vi "4Bar Arm Control.vi"(8 "Enable Setup":bool, 9 "4Bar Button":bool, 10 "Disable Sensor":bool, 11 "Joystick Input":dbl) -> ()   [LabVIEW 2014]
panel:
  out "Pot Error Out":errorcluster
  out "In Range?":bool
  out "PID Output":dbl format="%.2f"
  out "Output to Motor":dbl
  in  "Height Above Ground":dbl(slide)=0.40816326530612246 scale=0.2..0.8
  in  "PID gains":T1={"proportional gain (Kc)"=25.0, "integral time (Ti, min)"=0.015, "derivative time (Td, min)"=0.0}
  out "4Bar Pot Value":dbl
  out "Motor Output 4Bar":dbl(slide) scale=-1.0..1.0
  out "Motor Error Out":errorcluster
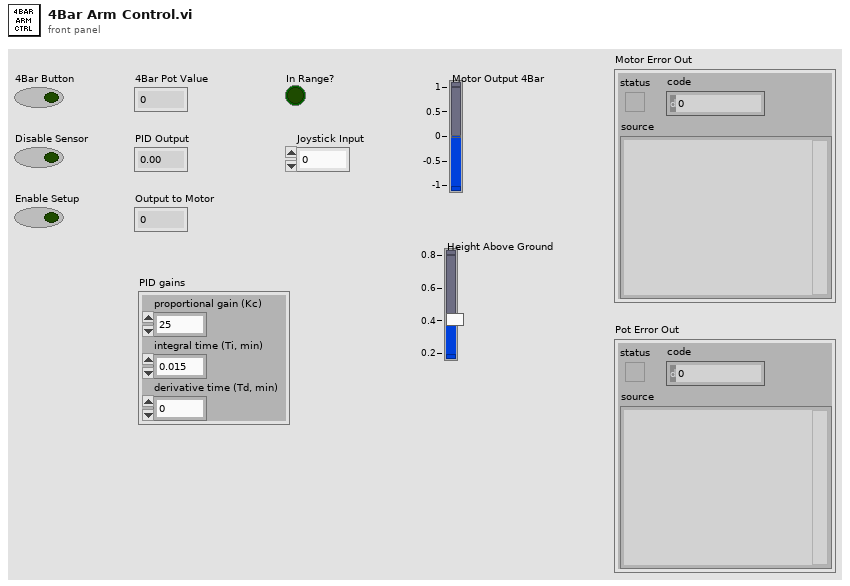
[diagram p1: front panel]
types:
  T1 = cluster{"proportional gain (Kc)":dbl, "integral time (Ti, min)":dbl, "derivative time (Td, min)":dbl}
  T2 = typedef "WPI_PotentiometerDevRef.ctl" = cluster{"DevStatus":errorcluster, "Controller":T3, "Analog Channel":T4, "Invert Output":bool}
  T3 = typedef "FPGA_TypedefAnalogModule.ctl" = enum16{"Controller 1"}
  T4 = typedef "FPGA_AIChannel.ctl" = enum8{"AI 0", "AI 1", "AI 2", "AI 3", "AI MXP 0", "AI MXP 1", "AI MXP 2", "AI MXP 3", "Invalid"}
  T5 = typedef "WPI_MotorControlDeviceRef.ctl" = cluster{"DeviceStatus":errorcluster, "Type":T6, "PWM":cluster{"Controller":T7, "PWM Channel":T8, "DeadBand":T9}, "CAN":cluster{"Device Number":u8, "Control Mode":T10, "Semaphore":T11, "Max Vout":dbl, "TalonSRX Control Mode":T12}, "Invert":bool, "TransformRef":T13, "InvTransformRef":T13}
  T6 = typedef "WPI_MotorControlType.ctl" = enum16{"PWM", "CAN", "CANTalonSRX"}
  T7 = typedef "FPGA_TypedefDigitalModule.ctl" = enum16{"Controller 1"}
  T8 = typedef "FPGA_DIOPWMChannel.ctl" = enum8{"PWM 0", "PWM 1", "PWM 2", "PWM 3", "PWM 4", "PWM 5", "PWM 6", "PWM 7", "PWM 8", "PWM 9", "PWM MXP 0", "PWM MXP 1", "PWM MXP 2", "PWM MXP 3", "PWM MXP 4", "PWM MXP 5", "PWM MXP 6", "PWM MXP 7", "PWM MXP 8", "PWM MXP 9", "Invalid"}
  T9 = typedef "WPI_PWMDeadband.ctl" = cluster{"Name":string, "maxPositivePwm":i32, "minPositivePwm":i32, "centerPwm":i32, "maxNegativePwm":i32, "minNegativePwm":i32, "angularRange":u16}
  T10 = typedef "WPI_CANJaguar_ControlMode.ctl" = enum8{"Percent VBus", "Current", "Speed", "Position", "Voltage"}
  T11 = typedef "Semaphore RefNum" = refnum<k1>
  T12 = typedef "WPI_CANTalonSRX_APIControlMode.ctl" = enum8{"Percent VBus", "Speed", "Position", "Slave", "Unchanged / Invalid"}
  T13 = typedef "WPI_PWMTransform_ConPane.ctl" = refnum<vi>
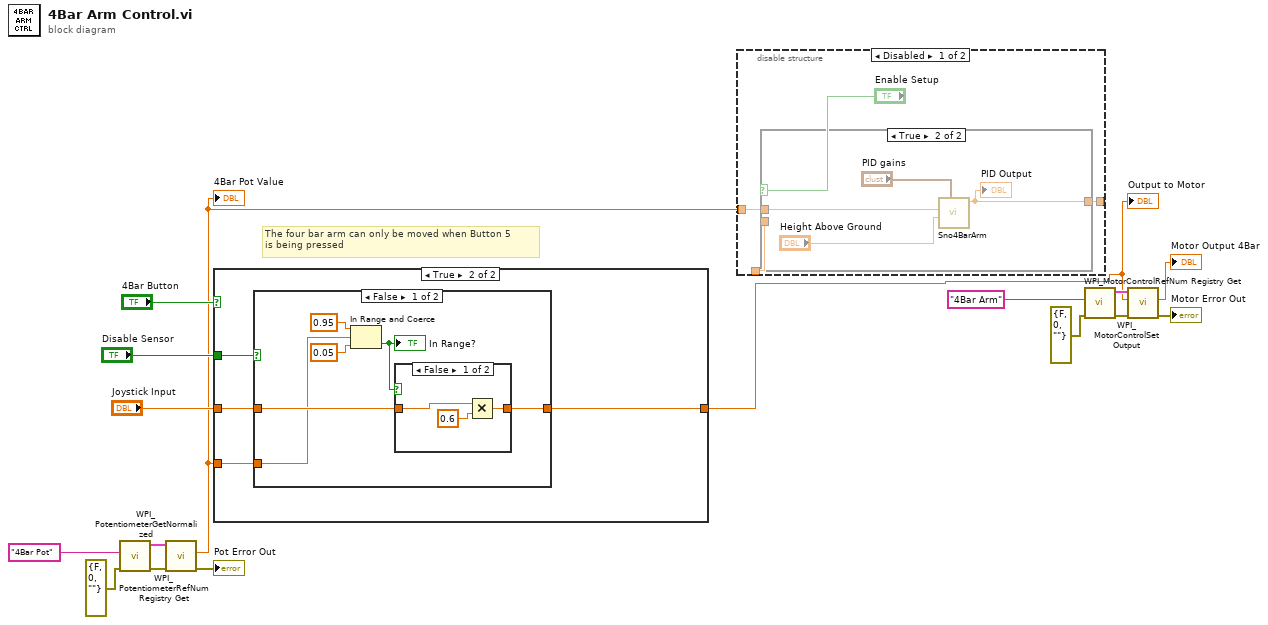
[diagram p0: block diagram]
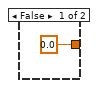
[diagram p4: hidden frame]
diagram:
  # "The four bar arm can only be moved when Button 5\nis being pressed"
  n1 = call <vilib>:"WPI_PotentiometerRefNum Registry Get.vi"("error in (no error)"=errorcluster {"status"=FALSE, "code"=0, "source"=""}, "refnum name"="4Bar Pot") -> ("error out"=w8:errorcluster, "PotDevRef"=w9:T2)  [unwired: 8 in]
  n2 = call <vilib>:"WPI_PotentiometerGetNormalized.vi"("error in"=w8, "PotDevRef"=w9) -> ("error out"=→"Pot Error Out":errorcluster, "Normalized Value"=w6:dbl)  [unwired: 7 in, 1 out]
  "4Bar Pot Value" <- w6
  n3 = case shown="True" "4Bar Button" {
    tunnel: "Joystick Input" -> [_ w21]
    tunnel: [0.0 ("Output") w20] -> w1
    tunnel: w6 -> [_ w19]
    tunnel: "Disable Sensor" -> [_ w18]
    frame False {
    }
    frame True {
      n4 = case shown="False" w18 {
        tunnel: w21 -> [w27 w32]
        tunnel: [w26 w32] -> w20
        tunnel: w19 -> [w23 _]
        frame False {
          n5 = In Range and Coerce(upper limit=0.95, x=w23, lower limit=0.05) -> (In Range?=w22:bool)  [unwired: 1 out]
          "In Range?" <- w22
          n6 = case shown="False" w22 {
            tunnel: w27 -> [w29 w31]
            tunnel: [w28 w31] -> w26
            frame False {
              n7 = Multiply(x=w29, y=0.6) -> (x*y=w28:dbl)
            }
            frame True {
            }
          }
        }
        frame True {
        }
      }
    }
  }
  "Output to Motor" <- w1
  n8 = disable-structure shown="Disabled" {
    disable-tunnel: w6 -> [w36 _]
    disable-tunnel: [w34 _] -> _
    disable-tunnel: _ -> [w33 _]
    frame Disabled {
      n9 = case shown="True" "Enable Setup" {
        tunnel: w36 -> [_ w39]
        tunnel: [w37 w38] -> w34
        tunnel: w33 -> [w37 _]
        frame False {
          # "When false just\npass the joystick\nvalue to the motor"
        }
        frame True {
          n10 = call "Sno4BarArm.vi"("Normalized Value"=w39, "Desired Height Above Ground"="Height Above Ground", "PID gains"="PID gains") -> ("output"=w38:dbl)  [unwired: 7 in]
          "PID Output" <- w38
        }
      }
    }
    frame Enabled {
    }
  }
  n11 = call <vilib>:"WPI_MotorControlRefNum Registry Get.vi"("error in (no error)"=errorcluster {"status"=FALSE, "code"=0, "source"=""}, "refnum name"="4Bar Arm") -> ("error out"=w11:errorcluster, "MotorControlDevRef"=w12:T5)  [unwired: 8 in]
  n12 = call <vilib>:"WPI_MotorControlSetOutput.vi"("error in (no error)"=w11, "Output"=w1, "MotorControlDevRef"=w12) -> ("error out"=→"Motor Error Out":errorcluster, "Motor Output"=→"Motor Output 4Bar":dbl)  [unwired: 6 in, 1 out]
